vi "PXIe-433x RT Driver VI.vi"(6 "Device Clock":string, 10 "Device Outputs FIFO":refnum<k33>, 11 "Device Reference":T1 format="%.0x") -> ()   [LabVIEW 2011, in "PXIe-433x Custom Device.lvlib"]
uses:
  PXIe-433x Custom Device.lvlib
  <vilib>/NI Veristand/Custom Device API/Custom Device Item Ref.ctl
  <vilib>/Platform/TimedLoop/XDataNode/timing_clust.ctl
  <vilib>/Platform/TimedLoop/XDataNode/nitl_modes.ctl
  <vilib>/Platform/TimedLoop/XDataNode/wakeup.ctl
  Global.vi
  <vilib>/NI Veristand/Custom Device API/Get Item Property (I32).vi
  <vilib>/NI Veristand/Custom Device API/Get Item Property (U32).vi
  <vilib>/Platform/TimedLoop/XDataNode/XDataNode.xnode
  <vilib>/Platform/TimedLoop/XDataNode/XDNodeRunTimeDep.lvlib
  <vilib>/NI Veristand/Custom Device API/Custom Device API.lvlib
  <vilib>/NI Veristand/Custom Device Tools/Custom Device Utility Library/Custom Device Utility Library.lvlib
panel:
  in  "Status Notifier":refnum<notifier>
  # "Custom Device Template\nv1.0"
  # "Use this template as a starting point for creating a custom device code module. The input controls shown here are specially named controls that the system will use to provide the device loop with data. The controls are not required for the device loop to run. For instance, if the device doesn't produce any output data, then you don't need the Device Outputs FIFO control. If you do use these controls, however, they need to have these exact names to be functional."
  # "The optional status notifier element is used to notify the RT engine of the last state of the custom device, and to indicate the device has completed execution. If this control is not used, a default No Error value is returned to the system when the device finishes execution.\n\nNote: This error state is not checked until the system shuts down. Use an output status channel to send more immediate status values to the system."
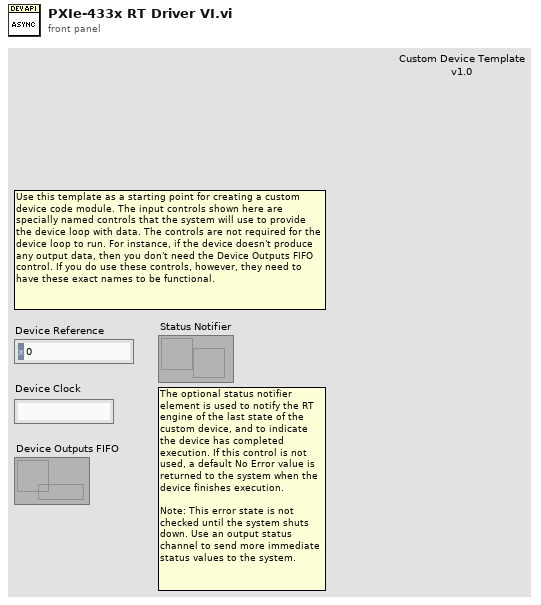
[diagram p1: front panel]
types:
  T1 = typedef "Custom Device API.lvlib/Custom Device Item Ref.ctl" = u64
  T2 = typedef "Custom Device API.lvlib/Custom Device Timed Loop Priority.ctl" = enum32{"Low", "Medium", "High"}
  T3 = typedef "XDNodeRunTimeDep.lvlib/timing_clust.ctl" = cluster{"Expected End [f-1]":u64, "Actual End [f-1]":u64, "Finished Late? [f-1]":bool, "Expected End [i-1]":u64, "Actual End [i-1]":u64, "Finished Late? [i-1]":bool, "Expected Start [i]":u64, "Actual Start [i]":u64, "Expected Start [f]":u64, "Actual Start [f]":u64, "Source Name":string, "Structure Name":string, "Period":i64, "Deadline":i64, "Offset":i64, "Start":i64, "Priority":i32, "Timeout":i32, "Mode":T4, "Wakeup Reason":T5, "Error":errorcluster, "Source Type":string, "Secondary Source Type":string, "Global End Time":u64, "Global Start Time":u64, "Frame Duration":u64, "Iteration Duration":u64, "Assigned CPU":i32, "I/O Scan Engine Mode":u32}
  T4 = typedef "XDNodeRunTimeDep.lvlib/nitl_modes.ctl" = enum32{"No Change", "Process missed periods, maintain original phase", "Discard missed periods, maintain original phase", "Process missed periods, ignore original phase", "Discard missed periods, ignore original phase"}
  T5 = typedef "XDNodeRunTimeDep.lvlib/wakeup.ctl" = enum32{"Normal", "Aborted", "Asynchronous wakeup", "Timing source error", "Timed loop error", "Timeout"}
  T6 = typedef "PXIe-433x Custom Device.lvlib/433x data.ctl" = cluster{"task":refnum<k21>, "Buffer":dbl[], "Started?":bool}
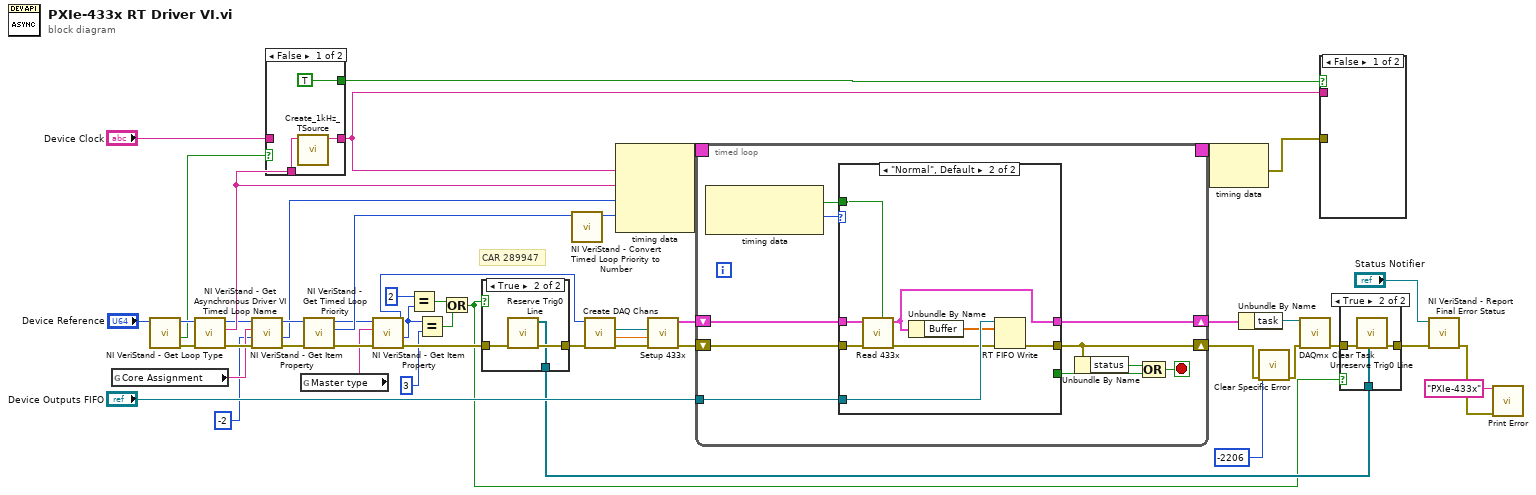
[diagram p0: block diagram]
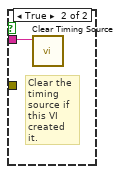
[diagram p4: hidden frame]
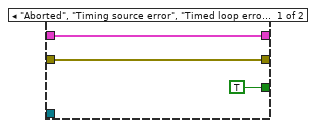
[diagram p6: hidden frame]
diagram:
  # "CAR 289947"
  n1 = global read "Global.vi" "Core Assignment"() -> (w8:string)
  n2 = call <vilib>:"NI VeriStand - Get Loop Type.vi"("Device Ref in"="Device Reference") -> ("error out"=w44:errorcluster, "Use Device Clock"=w41:bool, "Device Ref out"=w43:T1)  [unwired: 1 in, 7 out]
  n3 = call <vilib>:"NI VeriStand - Get Asynchronous Driver VI Timed Loop Name.vi"("error in (no error)"=w44, "Device Ref in"=w43) -> ("error out"=w12:errorcluster, "Device Timed Loop Name"=w23:string, "Device Ref out"=w10:T1)  [unwired: 7 out]
  n4 = call-poly <vilib>:"NI VeriStand - Get Item Property.vi"("error in (no error)"=w12, "Default Value"=-2, "Property Name"=w8, "Item Ref in"=w10) -> ("error out"=w11:errorcluster, "Value"=w7:i32, "Item Ref out"=w9:T1)  [unwired: 4 in, 1 out]
  n5 = case shown="False" w41 {
    tunnel: "Device Clock" -> [_ w53]
    tunnel: [w52 w53] -> w36
    tunnel: [TRUE _] -> w37
    tunnel: w23 -> [w50 _]
    frame False {
      n6 = call <vilib>:"Create_1kHz_TSource.vi"("name (in)"=w50) -> ("name (out)"=w52:string)  [unwired: 1 in, 9 out]
    }
    frame True {
    }
  }
  n7 = global read "Global.vi" "Master type"() -> (w20:string)
  n8 = call <vilib>:"NI VeriStand - Get Timed Loop Priority.vi"("error in (no error)"=w11, "Device Ref in"=w9) -> ("error out"=w22:errorcluster, "Priority"=w46:T2, "Device Ref out"=w21:T1)  [unwired: 7 out]
  n9 = call-poly <vilib>:"NI VeriStand - Get Item Property.vi"("error in (no error)"=w22, "Property Name"=w20, "Item Ref in"=w21) -> ("error out"=w18:errorcluster, "Value"=w2:u32, "Item Ref out"=w13:T1)  [unwired: 5 in, 1 out]
  n10 = Equal?(x=u32 2, y=w2) -> (x = y?=w5:bool)
  n11 = Equal?(x=w2, y=u32 3) -> (x = y?=w3:bool)
  n12 = Or(x=w5, y=w3) -> (x .or. y?=w4:bool)
  n13 = case shown="True" w4 {
    tunnel: w18 -> [w54 w57]
    tunnel: [w54 w56] -> w17
    tunnel: [_ w55] -> w14
    frame False {
    }
    frame True {
      n14 = call "Reserve Trig0 Line.vi"("error in (no error)"=w57) -> ("error out"=w56:errorcluster, "Backplane refs"=w55:refnum<visa-resource-name>[])  [unwired: 9 in]
    }
  }
  n15 = call <vilib>:"NI VeriStand - Convert Timed Loop Priority to Number.vi"("Priority"=w46) -> ("Numeric Priority"=w45:i32)  [unwired: 10 out]
  n16 = call "Create DAQ Chans.vi"("error in (no error)"=w17, "Device Reference"=w13) -> ("error out"=w25:errorcluster, "SampleRate"=w26:dbl, "task out"=w35:refnum<k21>)  [unwired: 6 in, 1 out]
  n17 = node-c288(w36, w23, w7, w45) -> (w48:T3)
  n18 = call "Setup 433x.vi"("error in (no error)"=w25, "SampleRate"=w26, "task in"=w35) -> ("error out"=w24:errorcluster, "433x"=w34:T6)  [unwired: 7 in]
  n19 = timed-loop {
    timing: w48 -> [_]
    timing-out: [_] -> w47
    shift-right: [w65] -> w28
    shift-left: w24 -> [w67]
    tunnel: "Device Outputs FIFO" -> [w66]
    shift-right: [w60] -> w31
    shift-left: w34 -> [w61]
    stop <- w62 stop-if-true
    n20 = node-c288() -> (w58:bool, w59:T5)  [unwired: 1 out]
    n21 = case shown="\"Normal\", Default" w59 {
      tunnel: w67 -> [w70 w72]
      tunnel: [w70 w75] -> w65
      tunnel: w66 -> [_ w78]
      tunnel: [TRUE _] -> w63
      tunnel: w61 -> [w68 w71]
      tunnel: [w68 w76] -> w60
      tunnel: w58 -> [_ w73]
      frame "Aborted", "Timing source error", "Timed loop error" {
      }
      frame "Normal", Default {
        n22 = call "Read 433x.vi"("Late?"=w73, "error in (no error)"=w72, "433x in"=w71) -> ("error out"=w77:errorcluster, "433x out"=w76:T6)  [unwired: 7 in]
        n23 = Unbundle By Name(w76) -> ("Buffer"=w74:dbl[])
        n24 = RT FIFO Write(0:w78, 1:w74, 3:w77) -> (11:w75:errorcluster)  [unwired: 1 in, 4 out]
      }
    }
    n25 = Unbundle By Name(w65) -> ("status"=w64:bool)
    n26 = Compound Arithmetic op=OR(w64, w63) -> (w62:bool)
  }
  n27 = node-c288(w47) -> (w38:errorcluster)
  n28 = Unbundle By Name(w31) -> ("task"=w30:refnum<k21>)
  n29 = call "Clear Specific Error.vi"("error in (no error)"=w28, "code"=-2206) -> ("error out"=w29:errorcluster)  [unwired: 9 in]
  n30 = call <vilib>:"DAQmx Clear Task.vi"("task in"=w30, "error in"=w29) -> ("error out"=w16:errorcluster)  [unwired: 13 in]
  n31 = case shown="False" w37 {
    tunnel: w38 -> [_ _]
    tunnel: w36 -> [_ w83]
    frame False {
    }
    frame True {
      # "Clear the timing source if this VI created it."
      n32 = call <vilib>:"Clear Timing Source.vi"("name"=w83) -> ()  [unwired: 1 in, 10 out]
    }
  }
  n33 = case shown="True" w4 {
    tunnel: w16 -> [w84 w87]
    tunnel: [w84 w86] -> w15
    tunnel: w14 -> [_ w85]
    frame False {
    }
    frame True {
      n34 = call "Unreserve Trig0 Line.vi"("Backplane refs"=w85, "error in (no error)"=w87) -> ("error out"=w86:errorcluster)  [unwired: 9 in]
    }
  }
  n35 = call <vilib>:"NI VeriStand - Report Final Error Status.vi"("error in (no error)"=w15, "Status Notifier"="Status Notifier") -> ("error out"=w33:errorcluster)  [unwired: 1 in, 8 out]
  n36 = call "Print Error.vi"("error out"=w33, "Your code's public name"="PXIe-433x") -> ()  [unwired: 9 in]
